vi "InitializeReport.vi"(8 "error in (no error)":errorcluster, 10 "Local Report Parameter":T1, 11 "LocalReport in":refnum<class "LocalReport.lvclass">) -> (0 "error out":errorcluster, 3 "LocalReport out":refnum<class "LocalReport.lvclass">)   [LabVIEW 2019, in "LocalReport.lvlib" / "LocalReport.lvclass"]
uses:
  LocalReport.lvclass
  LocalReport.lvclass/LocalReport.ctl
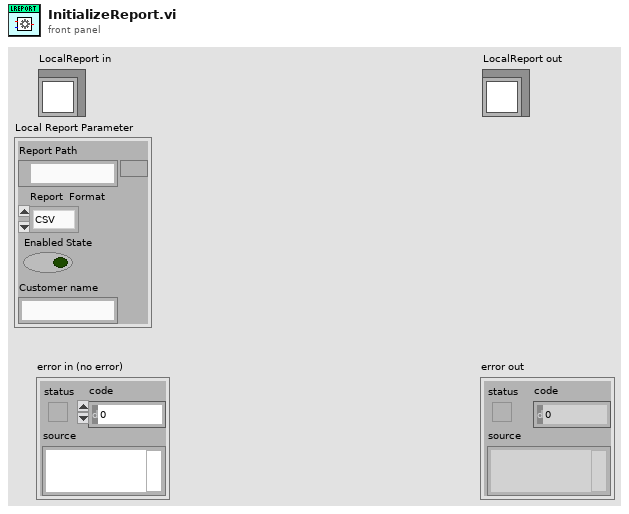
[diagram p1: front panel]
types:
  T1 = cluster{"Report Path":path, "Report  Format":enum16{"CSV", "XML", "PDF", "Excel", "TXT"}, "Enabled State":bool, "Customer name":string}
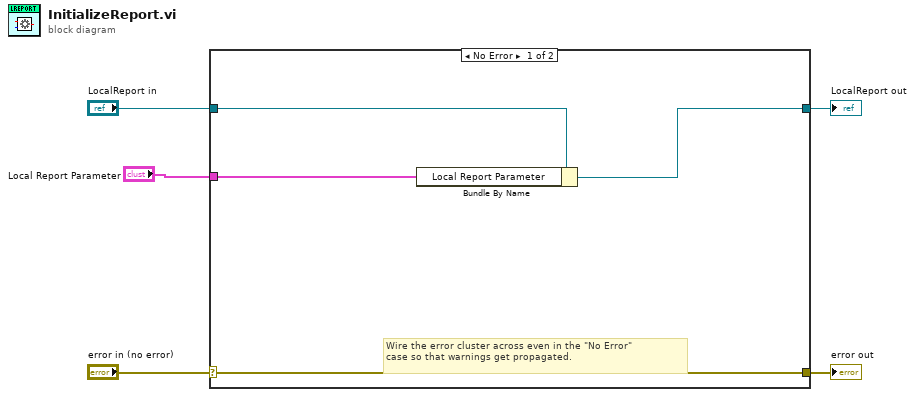
[diagram p0: block diagram]
diagram:
  n1 = case shown="No Error" "error in (no error)" {
    selector: "error in (no error)" -> [w9 w11]
    tunnel: [w9 w11] -> w4
    tunnel: [w7 w10] -> w2
    tunnel: "LocalReport in" -> [w8 w10]
    tunnel: "Local Report Parameter" -> [w6 _]
    frame No Error {
      # "Wire the error cluster across even in the \"No Error\"\ncase so that warnings get propagated."
      n2 = Bundle By Name(cluster=w8, "Local Report Parameter"=w6) -> (w7:refnum<class "LocalReport.lvclass">)
    }
    frame Error {
    }
  }
  "error out" <- w4
  "LocalReport out" <- w2
